vi "Configure Measurement Type.vi"(8 "error in (no error)":errorcluster, 10 "Measurement Type (0: Swept SA)":i32(ring) items=["Swept SA", "Channel Power", "Occupied Bandwidth", "Power Stat CCDF", "Adjacent Channel Power", "Burst Power", "Spurious Emissions", "Spectrum Emission Mask", "List Sweep", "TOI", "Harmonic"], 11 "VISA resource name":refnum<visa-resource-name>) -> (0 "error out":errorcluster, 3 "VISA resource name out":refnum<visa-resource-name>)   [LabVIEW 2014, in "Agilent MXA Series.lvlib"]
doc: "Selects the measurement type of the analyzer. Before you perform any measurement, you must call this VI to select the measurement type."
uses:
  Agilent MXA Series.lvlib
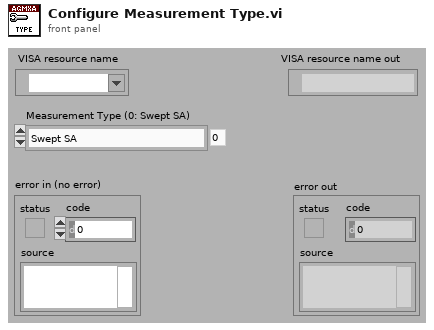
[diagram p1: front panel]
types:
  T1 = typedef "Agilent MXA Series.lvlib/Extended User Data.ctl" = cluster{"Measurement Type":i32, "Agilent MXA/EXA Model":i32}
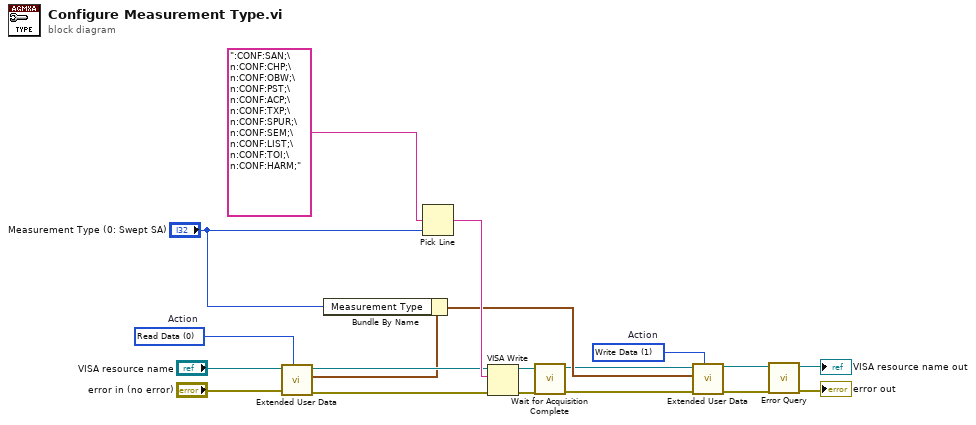
[diagram p0: block diagram]
diagram:
  w8 = 1 items=["Read Data", "Write Data", "Clear Data", "Clear ALL Data"]  # Action
  w13 = 0 items=["Read Data", "Write Data", "Clear Data", "Clear ALL Data"]  # Action
  n1 = call "Extended User Data.vi"("Action (1:Write Data)"=w13, "Error In (no error)"="error in (no error)", "VISA resource name in"="VISA resource name") -> ("Error Out"=w16:errorcluster, "User Data Out"=w1:T1, "VISA resource name out"=w17:refnum<visa-resource-name>)  [unwired: 6 in]
  n2 = Bundle By Name(cluster=w1, "Measurement Type"="Measurement Type (0: Swept SA)") -> (w11:T1)
  n3 = Pick Line(multi-line string=":CONF:SAN;\n:CONF:CHP;\n:CONF:OBW;\n:CONF:PST;\n:CONF:ACP;\n:CONF:TXP;\n:CONF:SPUR;\n:CONF:SEM;\n:CONF:LIST;\n:CONF:TOI;\n:CONF:HARM;", line index="Measurement Type (0: Swept SA)") -> (output string=w18:string)  [unwired: 1 in]
  n4 = VISA Write(VISA resource name=w17, write buffer=w18, error in (no error)=w16) -> (VISA resource name out=w14:refnum<visa-resource-name>, error out=w15:errorcluster)  [unwired: 1 out]
  n5 = call "Wait for Acquisition Complete.vi"("error in (no error)"=w15, "VISA resource name"=w14) -> ("error out"=w9:errorcluster, "VISA resource name out"=w10:refnum<visa-resource-name>)  [unwired: 8 in]
  n6 = call "Extended User Data.vi"("Action (1:Write Data)"=w8, "Error In (no error)"=w9, "User Data In"=w11, "VISA resource name in"=w10) -> ("Error Out"=w6:errorcluster, "VISA resource name out"=w7:refnum<visa-resource-name>)  [unwired: 5 in, 1 out]
  n7 = call "Error Query.vi"("error in (no error)"=w6, "VISA resource name"=w7) -> ("error out"=→"error out":errorcluster, "VISA resource name out"=→"VISA resource name out":refnum<visa-resource-name>)  [unwired: 6 in, 2 out]
